vi "processTelemetryUpdates.vi"   [LabVIEW 2015]
uses:
  <vilib>/rvi/Emulation/niFpgaGetClockAttributes.vi
  <vilib>/rvi/Emulation/niFpgaSctlEmulationGetInTimedLoop.vi
  <vilib>/rvi/Emulation/niFpgaEmulationReportErrorSimple.vi
  <vilib>/rvi/Emulation/niFpgaEmulationIsFPGAContextNoSignature.vi
  <vilib>/rvi/DataTransferAndStorage/Container/Common/niFpgaContainerGetUniqueNameForEmu.vi
  <vilib>/rvi/Memory/Memory_Emulation/niFpgaMemoryEmulationCacheClearOnFirstRun.vi
  <vilib>/rvi/Memory/Memory_Emulation/nirvimemoryEmulationManagerCache_MakeExclusive.vi
  <vilib>/rvi/Memory/Memory_Emulation/niFpgaMemoryEmulationValidateCache.vi
  <vilib>/rvi/Memory/Memory_Emulation/nirvimemoryEmulationManagerCache_InsertValue.vi
  <vilib>/Utility/error.llb/Clear Errors.vi
  <vilib>/rvi/Memory/Memory_Emulation/nirvimemoryEmulationManagerCache_ReleaseExclusive.vi
  <vilib>/rvi/Memory/Memory_Emulation/nirvimemoryEmulationManagerCache_GetValue.vi
  <vilib>/rvi/Memory/Memory_Emulation/nirvimemoryEmulationManagerCache_SetValue.vi
  <vilib>/rvi/Emulation/niFpgaProcessEmulError.vi
  <vilib>/rvi/errors/niFpgaSetErrorForExecOnDevCompSimple.vi
  <vilib>/rvi/eio/common/nirviEmuReportErrorAndStop.vi
  <vilib>/rvi/FIFO/Fifo_Resource/nirvififoEmulationSetSize.vi
  <vilib>/rvi/FIFO/Fifo_Resource/nirviFifoEmulationQueueMgr.vi
  <instcachedir>/0/nirviFifoEmulationQueueMgr_E5CAEC123FF24DC58D834DCA3CDAA9B5.lvgen/nirviFifoEmulationQueueMgr_E5CAEC123FF24DC58D834DCA3CDAA9B5_008.vi
  <vilib>/rvi/FIFO/Fifo_Resource/nirvififoEmulationCreateLock.vi
  <vilib>/rvi/FIFO/Fifo_Resource/nirvififoEmulationObtainLock.vi
  <vilib>/rvi/FIFO/Fifo_Resource/nirvififoEmulationReleaseLock.vi
  <vilib>/rvi/occurrence/nirviWaitOnOccurrenceBase.vi
  <vilib>/rvi/errors/nirviReportUnexpectedCaseInternalError.vi
  <vilib>/rvi/errors/nirviReportUnexpectedCaseInternalError (U32).vi
  <vilib>/rvi/Memory/Memory_Emulation/nirvimemoryFastEmulation.vi
  <vilib>/rvi/Memory/Memory_Emulation/nirvimemoryEmulation.vi
  <vilib>/rvi/Emulation/niFpgaCriticalErrorInLSC.vi
  <vilib>/rvi/DataTransferAndStorage/Container/XNode/niFpgaContainer.xnode
  <vilib>/rvi/DataTransferAndStorage/Register/Emulation/niFpgaRegisterEmulation.vi
  <vilib>/rvi/FIFO/Fifo_Resource/nirvififoEmulationRead.vi
types:
  T1 = cluster{"Address":u32, "Telemetry Update Mode":enum8{"NOP", "Set", "Add", "Subtract", "Or"}, "Data":u32}
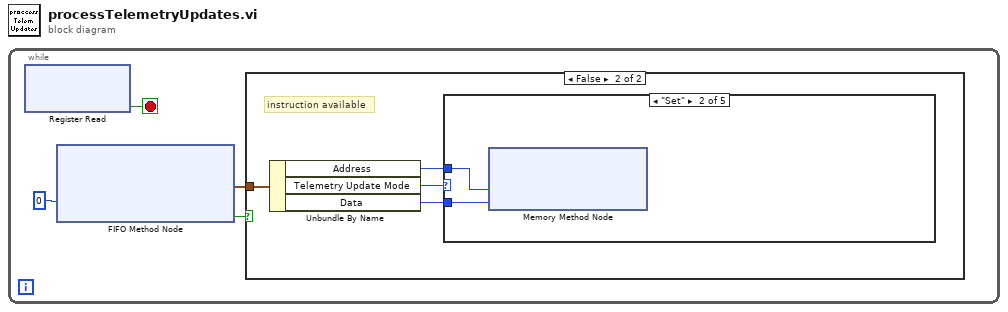
[diagram p0: block diagram]
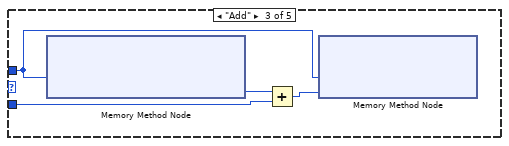
[diagram p4: hidden frame]
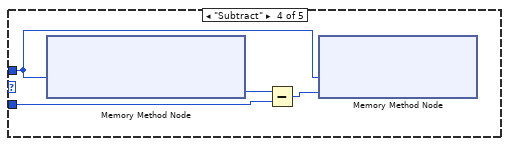
[diagram p5: hidden frame]
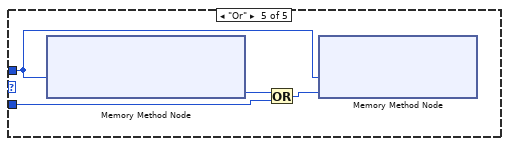
[diagram p6: hidden frame]
diagram:
  n1 = while {
    stop <- w4 stop-if-true
    n2 = xnode ("Register Read")() -> ("Data"=w4:bool)  [unwired: 1 in, 1 out]
    n3 = xnode ("FIFO Method Node")("Timeout"=0) -> ("Element"=w1:T1, "Timed Out?"=w2:bool)  [unwired: 1 in, 1 out]
    n4 = case shown="False" w2 {
      tunnel: w1 -> [_ w8]
      frame True {
        # "no instruction available"
      }
      frame False {
        # "instruction available"
        n5 = Unbundle By Name(w8) -> ("Address"=w6:u32, "Telemetry Update Mode"=w7:enum8{"NOP", "Set", "Add", "Subtract", "Or"}, "Data"=w5:u32)
        n6 = case shown="\"Set\"" w7 {
          tunnel: w6 -> [_ w10 w13 w17 w21]
          tunnel: w5 -> [_ w9 w11 w15 w19]
          frame "NOP", Default {
          }
          frame "Set" {
            n7 = xnode ("Memory Method Node")("Address"=w10, "Data"=w9) -> ()  [unwired: 1 in, 1 out]
          }
          frame "Add" {
            n8 = xnode ("Memory Method Node")("Address"=w13) -> ("Data"=w14:u32)  [unwired: 1 in, 1 out]
            n9 = Add(x=w14, y=w11) -> (x+y=w12:u32)
            n10 = xnode ("Memory Method Node")("Address"=w13, "Data"=w12) -> ()  [unwired: 1 in, 1 out]
          }
          frame "Subtract" {
            n11 = xnode ("Memory Method Node")("Address"=w17) -> ("Data"=w18:u32)  [unwired: 1 in, 1 out]
            n12 = Subtract(x=w18, y=w15) -> (x-y=w16:u32)
            n13 = xnode ("Memory Method Node")("Address"=w17, "Data"=w16) -> ()  [unwired: 1 in, 1 out]
          }
          frame "Or" {
            n14 = xnode ("Memory Method Node")("Address"=w21) -> ("Data"=w22:u32)  [unwired: 1 in, 1 out]
            n15 = Or(x=w22, y=w19) -> (x .or. y?=w20:u32)
            n16 = xnode ("Memory Method Node")("Address"=w21, "Data"=w20) -> ()  [unwired: 1 in, 1 out]
          }
        }
      }
    }
  }
